vi "CaptureImage(Async).vi"(6 "timeout in ms (5000)":i32=5000, 8 "error in (no error)":errorcluster, 11 "Microscope":refnum<class "Microscope.lvclass">) -> (0 "error out":errorcluster, 2 "buffer":i32, 3 "Microscope out":refnum<class "Microscope.lvclass">)   [LabVIEW 2015, in "Microscope.lvclass"]
doc: "---------------------------------------------------------------\nJKI State Machine Objects™\nhttp://jki.net/state-machine-objects/\nCopyright (C) 2005-2015, JKI <info@jki.net>\nALL RIGHTS RESERVEDJKI State Machine Objects (SMO) 1.0.0.4\nJKI - JKI\nCopyright (c) 2015, JKI"
uses:
  Microscope.lvclass
  Microscope.lvclass/Microscope.ctl
  Typedefs/PrivateEvents--Microscope.CaptureImageAtPosition.ctl
  XYStage/Typedefs/(real)Coords--Cluster.ctl
  XYStage/XYStage.lvclass
panel:
  # "For instructions on how to use the JKI State Machine Objects, examples and video tutorials, visit:\nhttp://jki.net/state-machine-objects/\n\nJKI State Machine Objects™\nhttp://jki.net/state-machine-objects/\nCopyright (C) 2005-2015, JKI <info@jki.net>\nALL RIGHTS RESERVED"
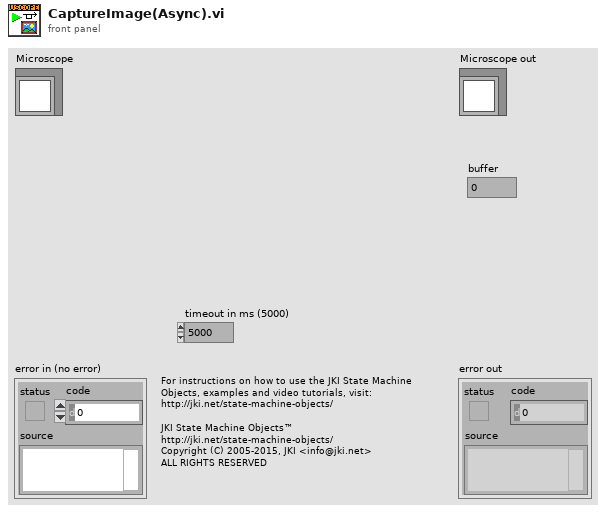
[diagram p1: front panel]
types:
  T1 = typedef "Microscope.lvclass/PrivateEvents--Microscope.CaptureImageAtPosition.ctl" = cluster{"Coords":T2, "image notifier":refnum<notifier>, "Move?":bool}
  T2 = typedef "XYStage.lvclass/(real)Coords--Cluster.ctl" = cluster{"X":dbl, "Y":dbl}
  T3 = typedef "Microscope.lvclass/PrivateData--Ref.ctl" = refnum<data-value>
  T4 = typedef "Microscope.lvclass/PrivateData--Cluster.ctl" = cluster{"Public Events":T5, "Protected Events":T6, "Private Events":T7, "Dependencies":T8, "Configuration":T9}
  T5 = typedef "Microscope.lvclass/PublicEvents--Cluster.ctl" = cluster{"Value Changed":refnum<user-event>, "Initialized":refnum<user-event>}
  T6 = typedef "Microscope.lvclass/ProtectedEvents--Cluster.ctl" = cluster{"placeholder":refnum<user-event>}
  T7 = typedef "Microscope.lvclass/PrivateEvents--Cluster.ctl" = cluster{"New Value":refnum<user-event>, "Initialize":refnum<user-event>, "CaptureImageAtPosition":refnum<user-event>}
  T8 = typedef "Microscope.lvclass/Dependencies--Cluster.ctl" = cluster{"XYStage":refnum<class "XYStage.lvclass">, "Camera":refnum<class "Camera.lvclass">}
  T9 = typedef "Microscope.lvclass/Configuration--Cluster.ctl" = cluster{"XY Stage":string, "Camera":string, "image output folder":path, "filetype":string}
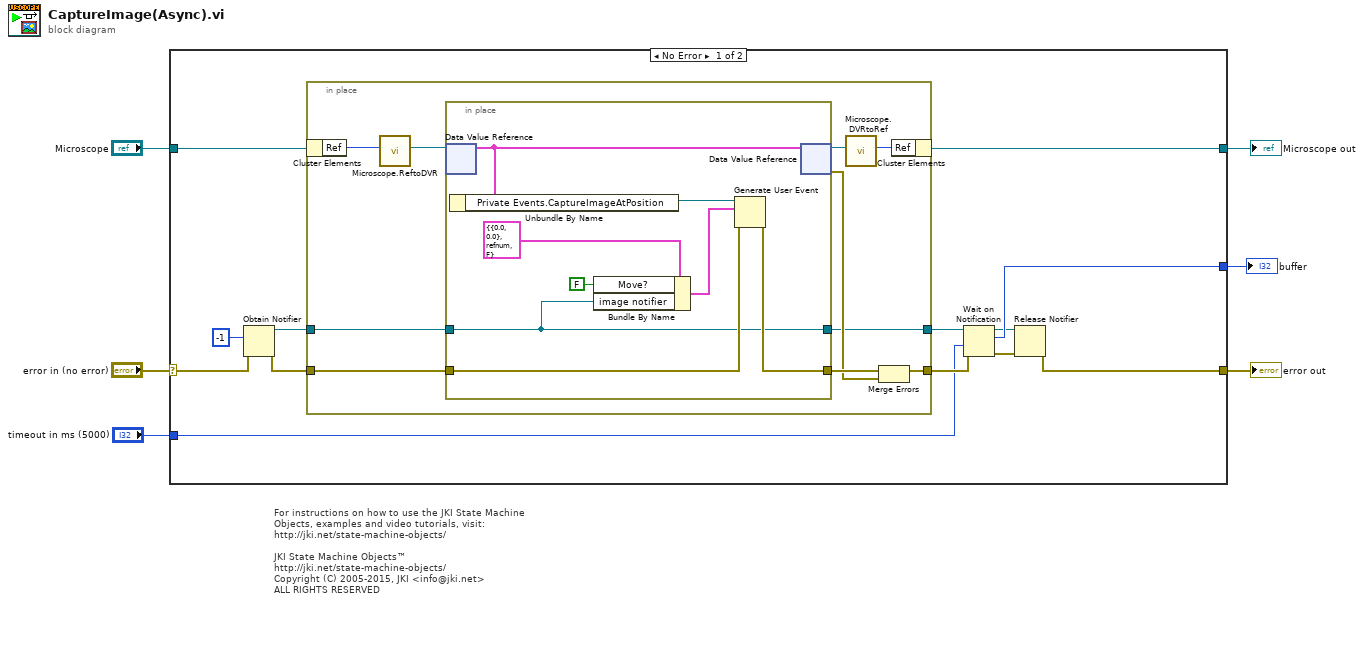
[diagram p0: block diagram]
diagram:
  # "For instructions on how to use the JKI State Machine Objects, examples and video tutorials, visit:\nhttp://jki.net/state-machine-objects/\n\nJKI State Machine Objects™\nhttp://jki.net/state-machine-objects/\nCopyright (C) 2005-2015, JKI <info@jki.net>\nALL RIGHTS RESERVED"
  n1 = case shown="No Error" "error in (no error)" {
    selector: "error in (no error)" -> [w15 w39]
    tunnel: [w9 w39] -> w5
    tunnel: [w18 w38] -> w6
    tunnel: "Microscope" -> [w19 w38]
    tunnel: [w11 _] -> w2
    tunnel: "timeout in ms (5000)" -> [w7 _]
    frame No Error {
      n2 = Obtain Notifier(notification data type=-1 ("buffer"), error in (no error)=w15) -> (notifier out=w16:refnum<notifier>, error out=w14:errorcluster)  [unwired: 2 in, 1 out]
      n3 = in-place {
        in-place-border: w14 -> [w29]
        in-place-border: [w26] -> w8
        in-place-border: w16 -> [w21]
        in-place-border: [w20] -> w13
        n4 = in-place-cluster #1(w19) -> ("Ref"=w25:u32)
        n5 = call "Microscope.ReftoDVR.vi"("Ref"=w25) -> ("Ref"=w23:T3)  [unwired: 10 in]
        n6 = in-place {
          in-place-border: w29 -> [w35]
          in-place-border: [w34] -> w28
          in-place-border: w21 -> [w32]
          in-place-border: [w32] -> w20
          n7 = in-place-dvr #2(w23) -> (w37:T4)  [unwired: 1 out]
          n8 = Unbundle By Name(w37) -> ("Private Events.CaptureImageAtPosition"=w36:refnum<user-event>)
          n9 = Bundle By Name(cluster=T1 {"Coords"={"X"=0.0, "Y"=0.0}, "image notifier"=refnum, "Move?"=FALSE} ("CaptureImageAtPosition"), "Move?"=FALSE, "image notifier"=w32) -> (w31:T1)
          n10 = Generate User Event(user event=w36, event data cluster=w31, error in=w35) -> (error out=w34:errorcluster)  [unwired: 1 in, 1 out]
          n11 = in-place-dvr #2(w37) -> (w24:T3, w27:errorcluster)
        }
        n12 = call "Microscope.DVRtoRef.vi"("Ref"=w24) -> ("Ref"=w22:u32)  [unwired: 10 in]
        n13 = Merge Errors(w28, w27) -> (w26:errorcluster)
        n14 = in-place-cluster #1("Ref"=w22) -> (w18:refnum<class "Microscope.lvclass">)
      }
      n15 = Wait on Notification(notifier=w13, timeout in ms (-1)=w7, error in (no error)=w8) -> (notifier out=w10:refnum<notifier>, notification=w11:i32, error out=w12:errorcluster)  [unwired: 1 in, 1 out]
      n16 = Release Notifier(notifier=w10, error in (no error)=w12) -> (error out=w9:errorcluster)  [unwired: 1 in, 2 out]
    }
    frame Error {
    }
  }
  "error out" <- w5
  "Microscope out" <- w6
  "buffer" <- w2
